vi "Update Buttons.vi"(8 "error in (no error)":errorcluster, 11 "GripsMaster in":refnum<class "GripsMaster.lvclass">) -> (0 "error out":errorcluster, 3 "GripsMaster out":refnum<class "GripsMaster.lvclass">)   [LabVIEW 2013, in "GripsMaster.lvclass"]
uses:
  GripsMaster.lvclass
  GripsMaster.lvclass/GripsMaster.ctl
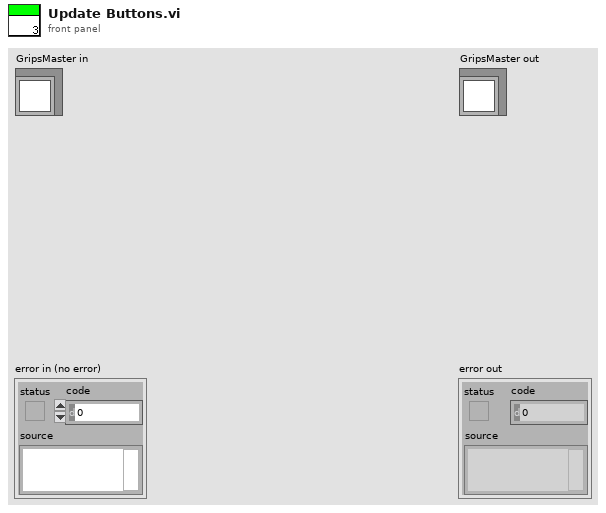
[diagram p1: front panel]
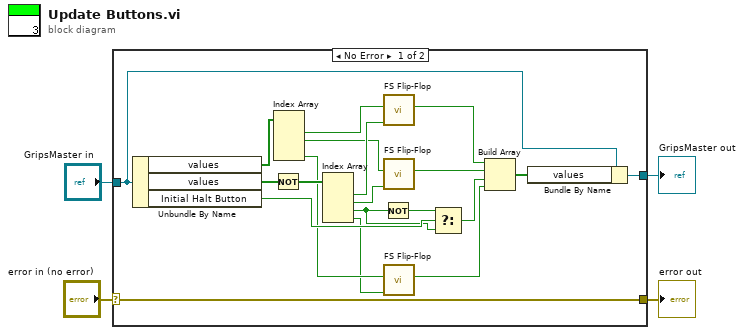
[diagram p0: block diagram]
diagram:
  n1 = case shown="No Error" "error in (no error)" {
    selector: "error in (no error)" -> [w24 w26]
    tunnel: [w24 w26] -> w3
    tunnel: [w22 w25] -> w1
    tunnel: "GripsMaster in" -> [w21 w25]
    frame No Error {
      n2 = Unbundle By Name(w21) -> ("values"=w14:bool[], "values"=w23:bool[], "Initial Halt Button"=w17:bool)
      n3 = Not(x=w23) -> (.not. x?=w19:bool[])
      n4 = Index Array(array=w14) -> (element #1=w13:bool, element #2=w10:bool, element #4=w7:bool)  [unwired: 4 in, 1 out]
      n5 = Index Array(array=w19) -> (element #1=w15:bool, element #2=w9:bool, element #3=w16:bool, element #4=w6:bool)  [unwired: 4 in]
      n6 = Not(x=w16) -> (.not. x?=w20:bool)
      n7 = call "FS Flip-Flop.vi"("Button Value"=w15, "Current State"=w13) -> ("result"=w12:bool)  [unwired: 9 in]
      n8 = call "FS Flip-Flop.vi"("Button Value"=w9, "Current State"=w10) -> ("result"=w11:bool)  [unwired: 9 in]
      n9 = call "FS Flip-Flop.vi"("Button Value"=w6, "Current State"=w7) -> ("result"=w8:bool)  [unwired: 9 in]
      n10 = Select(t=w20, s=w17, f=w16) -> (s? t:f=w18:bool)
      n11 = Build Array(w12, w11, w18, w8) -> (w5:bool[])
      n12 = Bundle By Name(cluster=w21, "values"=w5) -> (w22:refnum<class "GripsMaster.lvclass">)
    }
    frame Error {
    }
  }
  "error out" <- w3
  "GripsMaster out" <- w1
